vi "test user button.vi"() -> ()   [LabVIEW 2016]
uses:
  <vilib>/NI_Real-Time Target Support.lvlib
panel:
  out "Boolean 5":bool
  out "Boolean 4":bool
  out "Boolean 3":bool
  out "Boolean 2":bool
  out "Boolean":bool
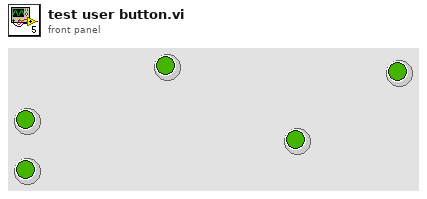
[diagram p1: front panel]
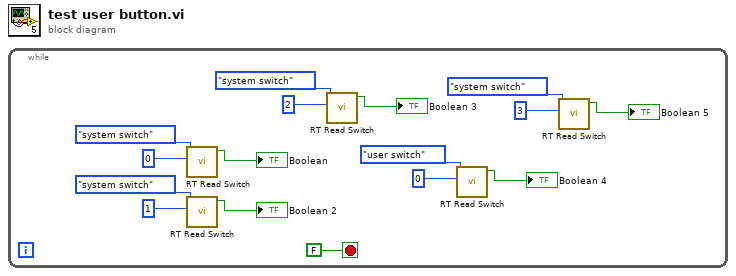
[diagram p0: block diagram]
diagram:
  n1 = while {
    stop <- FALSE stop-if-true
    n2 = call <vilib>:"RT Read Switch.vi"("switch ID"=0, "switch type (system switch)"=enum16{"system switch", "user switch"}."system switch") -> ("switch state (on/off)"=→"Boolean":bool)  [unwired: 8 in, 1 out]
    n3 = call <vilib>:"RT Read Switch.vi"("switch ID"=1, "switch type (system switch)"=enum16{"system switch", "user switch"}."system switch") -> ("switch state (on/off)"=→"Boolean 2":bool)  [unwired: 8 in, 1 out]
    n4 = call <vilib>:"RT Read Switch.vi"("switch ID"=2, "switch type (system switch)"=enum16{"system switch", "user switch"}."system switch") -> ("switch state (on/off)"=→"Boolean 3":bool)  [unwired: 8 in, 1 out]
    n5 = call <vilib>:"RT Read Switch.vi"("switch ID"=0, "switch type (system switch)"=enum16{"system switch", "user switch"}."user switch") -> ("switch state (on/off)"=→"Boolean 4":bool)  [unwired: 8 in, 1 out]
    n6 = call <vilib>:"RT Read Switch.vi"("switch ID"=3, "switch type (system switch)"=enum16{"system switch", "user switch"}."system switch") -> ("switch state (on/off)"=→"Boolean 5":bool)  [unwired: 8 in, 1 out]
  }
